vi "Main.vi"() -> ()   [LabVIEW 2020]
panel:
  out "x * y":dbl
  in  "y":dbl=8.0
  in  "x":dbl=9.0
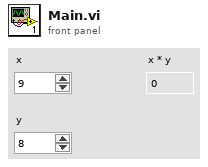
[diagram p1: front panel]
types:
  T1 = enum32{"invalid app kind", "Development System", "Run Time System", "Student Edition", "Embedded LabVIEW", "Evaluation", "Custom"}
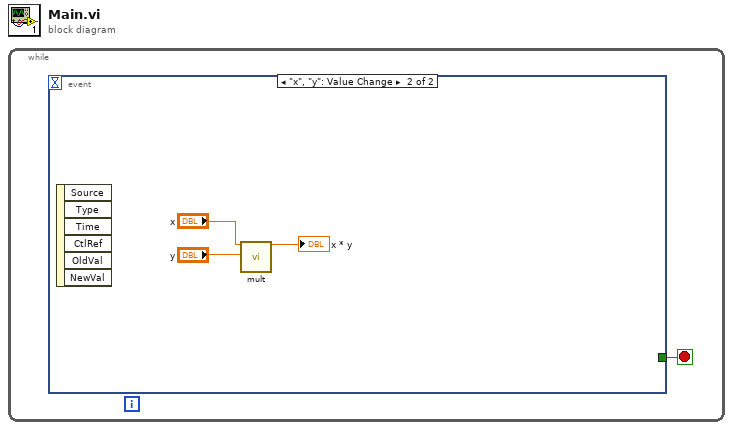
[diagram p0: block diagram]
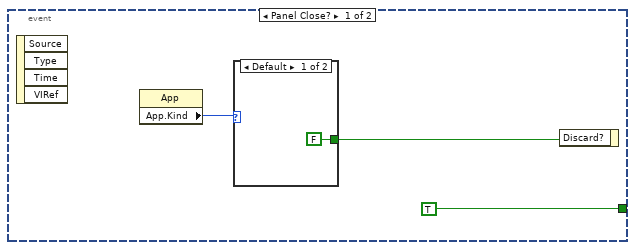
[diagram p2: hidden frame]
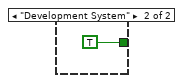
[diagram p3: hidden frame]
diagram:
  n1 = while {
    stop <- w1 stop-if-true
    n2 = event shown="[1] \"x\", \"y\": Value Change" {
      selector: _ -> [_ _]
      dyn-events: _ -> [_ _]
      timeout: _ -> [_ _]
      tunnel: [TRUE _] -> w1
      event Panel Close? {
        n3 = event-data() -> ()  [unwired: 1 in, 4 out]
        n4 = property class="App"() -> ("App.Kind"=w3:T1)  [unwired: 2 in, 2 out]
        n5 = case shown="Default" w3 {
          tunnel: [FALSE TRUE] -> w2
          frame Default {
          }
          frame "Development System" {
          }
        }
        n6 = event-data("Discard?"=w2) -> ()  [unwired: 1 in, 1 out]
      }
      event "x", "y": Value Change {
        n7 = event-data() -> ()  [unwired: 1 in, 6 out]
        n8 = call "mult.vi"("x"="x", "y"="y") -> ("x*y"=→"x * y":dbl)  [unwired: 16 in, 1 out]
      }
    }
  }
